vi "VSG_SET_RF_STATE_1.00.vi"(4 "RF ON/OFF (OFF)":bool, 6 "Delay Time (ms)":dbl=1.0 caption="Delay Time (s)", 7 "RO(t)":bool, 8 "error in":errorcluster {"code" format="%.0x"}, 11 "Session In":refnum<visa-resource-name>="TCPIP0::169.254.70.100::inst0::INSTR") -> (0 "error out":errorcluster {"code" format="%.0x"}, 3 "Session Out":refnum<visa-resource-name>="TCPIP0::169.254.70.100::inst0::INSTR", 5 "rf_on(t)":bool)   [LabVIEW 2018]
doc: "Launches the Instrument I/O Assistant, which you can use to communicate with message-based instruments and graphically parse the response. For example you can communicate with an instrument that uses a serial, Ethernet, or GPIB interface."
panel:
  in  "Timeout":u32=3000
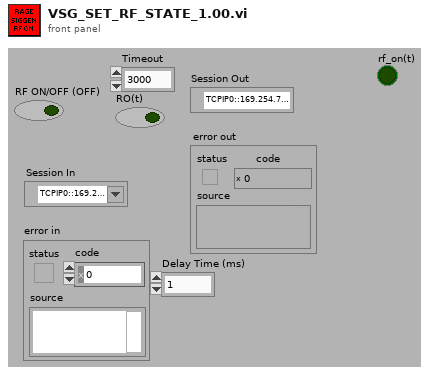
[diagram p1: front panel]
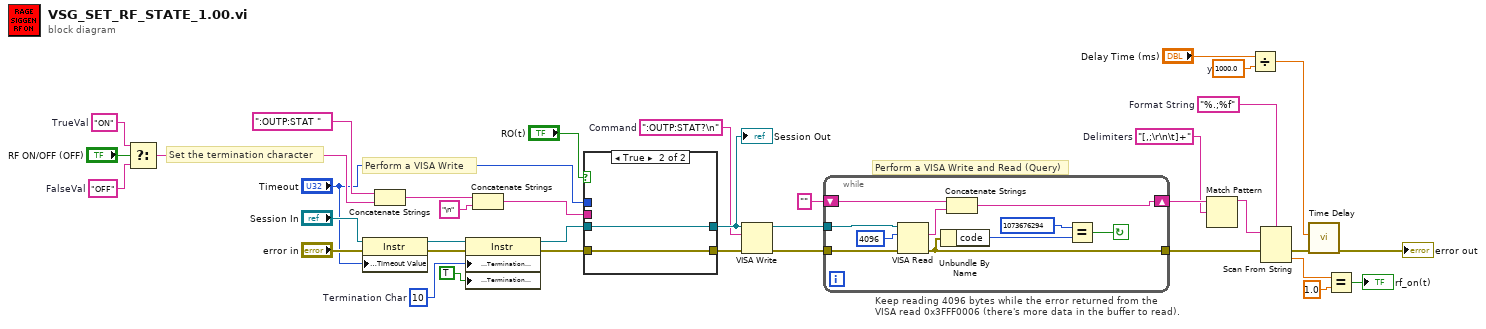
[diagram p0: block diagram]
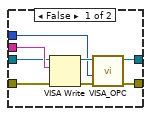
[diagram p2: hidden frame]
diagram:
  w10 = "[,;\r\n\t]+"  # Delimiters
  w11 = "%.;%f"  # Format String
  w1 = ":OUTP:STAT?\n"  # Command
  w18 = 1000.0  # y
  w28 = u8 10  # Termination Char
  w34 = "OFF"  # FalseVal
  w35 = "ON"  # TrueVal
  # "Perform a VISA Write and Read (Query)"
  # "Keep reading 4096 bytes while the error returned from the\nVISA read 0x3FFF0006 (there's more data in the buffer to read)."
  # "Perform a VISA Write"
  # "Set the termination character"
  n1 = Select(t=w35, s="RF ON/OFF (OFF)", f=w34) -> (s? t:f=w33:string)
  n2 = property class="Instr"(reference="Session In", error in="error in", "General Settings:Timeout Value"="Timeout") -> (reference out=w31:refnum<visa-resource-name>, error out=w30:errorcluster)
  n3 = Concatenate Strings(":OUTP:STAT " ("staticText"), w33) -> (w26:string)
  n4 = property class="Instr"(reference=w31, error in=w30, "Message Based Settings:Termination Character"=w28, "Message Based Settings:Termination Character Enable"=TRUE ("enable")) -> (reference out=w22:refnum<visa-resource-name>, error out=w29:errorcluster)
  n5 = Concatenate Strings(w26, "\n" ("StaticText")) -> (w24:string)
  n6 = case shown="True" "RO(t)" {
    tunnel: w29 -> [w45 w46]
    tunnel: w24 -> [w44 _]
    tunnel: [w43 w46] -> w7
    tunnel: w22 -> [w42 w47]
    tunnel: [w41 w47] -> w6
    tunnel: "Timeout" -> [w38 _]
    frame False {
      n7 = VISA Write(VISA resource name=w42, write buffer=w44, error in (no error)=w45) -> (VISA resource name out=w39:refnum<visa-resource-name>, error out=w40:errorcluster)  [unwired: 1 out]
      n8 = call "VISA_OPC.vi"("error in"=w40, "Timeout"=w38, "Session In"=w39) -> ("error out"=w43:errorcluster, "Session Out"=w41:refnum<visa-resource-name>)  [unwired: 6 in, 1 out]
    }
    frame True {
    }
  }
  "Session Out" <- w6
  n9 = VISA Write(VISA resource name=w6, write buffer=w1, error in (no error)=w7) -> (VISA resource name out=w17:refnum<visa-resource-name>, error out=w16:errorcluster)  [unwired: 1 out]
  n10 = while {
    tunnel: w17 -> [w54]
    shift-right: [w48] -> w13
    shift-left: "" -> [w53]
    tunnel: w16 -> [w51]
    tunnel: [w50] -> w15
    stop <- w49 continue-if-true
    n11 = VISA Read(VISA resource name=w54, byte count=u32 4096 ("byte count (0)"), error in (no error)=w51) -> (read buffer=w52:string, error out=w50:errorcluster)  [unwired: 2 out]
    n12 = Unbundle By Name(w50) -> ("code"=w56:i32)
    n13 = Concatenate Strings(w53, w52) -> (w48:string)
    n14 = Equal?(x=1073676294, y=w56) -> (x = y?=w49:bool)
  }
  n15 = Match Pattern(string=w13, regular expression=w10) -> (before substring=w12:string)  [unwired: 1 in, 3 out]
  n16 = Divide(x="Delay Time (ms)", y=w18) -> (x/y=w20:dbl)
  n17 = Scan From String(format string=w11, input string=w12, error in=w15) -> (error out=w5:errorcluster, output 1=w4:dbl)  [unwired: 2 in, 2 out]
  n18 = call "Time Delay"("error in (no error)"=w5, "Delay Time (s)"=w20) -> ("error out"=→"error out":errorcluster)  [unwired: 9 in]
  n19 = Equal?(x=w4, y=1.0) -> (x = y?=→"rf_on(t)":bool)
